vi "Calculate matching sides.vi"(8 "error in (no error)":errorcluster, 11 "Tile in":refnum<class "Tile.lvclass">) -> (0 "error out":errorcluster, 3 "Tile out":refnum<class "Tile.lvclass">)   [LabVIEW 2020, in "Tile.lvclass"]
uses:
  Tile.lvclass
  Tile.lvclass/Tile.ctl
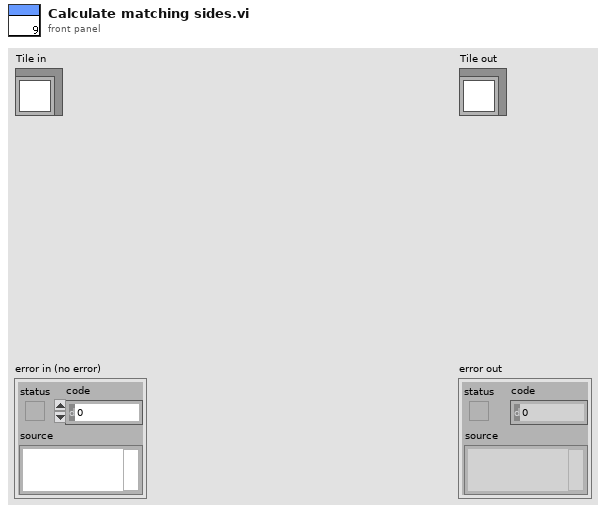
[diagram p1: front panel]
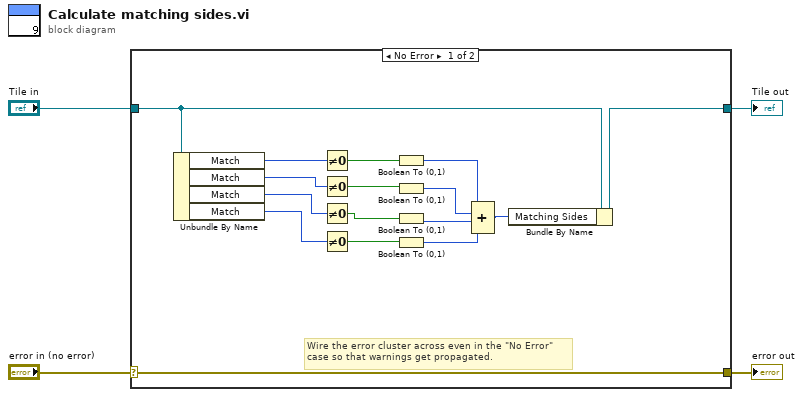
[diagram p0: block diagram]
diagram:
  n1 = case shown="No Error" "error in (no error)" {
    selector: "error in (no error)" -> [w20 w22]
    tunnel: [w20 w22] -> w3
    tunnel: [w10 w21] -> w1
    tunnel: "Tile in" -> [w9 w21]
    frame No Error {
      # "Wire the error cluster across even in the \"No Error\"\ncase so that warnings get propagated."
      n2 = Unbundle By Name(w9) -> ("Match"=w19:u64, "Match"=w17:u64, "Match"=w18:u64, "Match"=w16:u64)
      n3 = Not Equal To 0?(x=w19) -> (x != 0?=w8:bool)
      n4 = Not Equal To 0?(x=w17) -> (x != 0?=w7:bool)
      n5 = Not Equal To 0?(x=w18) -> (x != 0?=w6:bool)
      n6 = Not Equal To 0?(x=w16) -> (x != 0?=w5:bool)
      n7 = Boolean To (0,1)(Boolean=w8) -> (0, 1=w12:i16)
      n8 = Boolean To (0,1)(Boolean=w7) -> (0, 1=w13:i16)
      n9 = Boolean To (0,1)(Boolean=w6) -> (0, 1=w14:i16)
      n10 = Boolean To (0,1)(Boolean=w5) -> (0, 1=w15:i16)
      n11 = Compound Arithmetic op=ADD(w12, w13, w14, w15) -> (w11:i16)
      n12 = Bundle By Name(cluster=w9, "Matching Sides"=w11) -> (w10:refnum<class "Tile.lvclass">)
    }
    frame Error {
    }
  }
  "error out" <- w3
  "Tile out" <- w1
